vi "Pre Launch Init.vi"(11 "Nested in":refnum<class "Paquetes.lvclass">) -> (0 "error out":errorcluster, 3 "Nested out":refnum<class "Paquetes.lvclass">)   [LabVIEW 2020, in "Paquetes.lvlib" / "Paquetes.lvclass"]
doc: "(<B>Filename</B>: Actor Framework.lvlib:Actor.lvclass:Pre Launch Init.vi)\n\nDefines behavior that occurs after the Launch Nested Actor method is invoked but before the actor's Actor Core method begins running.\n\nBy default, this method does nothing. A descendant class may override it to define behavior."
uses:
  Paquetes.lvclass
  C:/Program Files (x86)/National Instruments/LabVIEW 2020/vi.lib/ActorFramework/Actor/Actor.lvclass
  Paquetes.lvclass/Paquetes.ctl
  <vilib>/ActorFramework/Actor/Actor.lvclass/Actor.ctl
  <vilib>/ActorFramework/Message Enqueuer/Message Enqueuer.lvclass/Message Enqueuer.ctl
  <vilib>/ActorFramework/Message Enqueuer/Enqueue.vi
  <vilib>/ActorFramework/Message Enqueuer/Init from Existing Queue.vi
  Paquetes Messages/DRAW FP PAQUETES IN UI Msg/DRAW FP PAQUETES IN UI Msg.lvclass
  C:/Program Files (x86)/National Instruments/LabVIEW 2020/vi.lib/ActorFramework/Message/Message.lvclass
  <vilib>/ActorFramework/Message Priority Queue/Priority Enqueue.vi
  <vilib>/ActorFramework/Message Enqueuer/Message Enqueuer.lvclass
  <vilib>/ActorFramework/Actor/Actor.lvclass
  C:/Users/HP/Desktop/Salma_Aguayo/Paquetes/Paquetes.lvclass
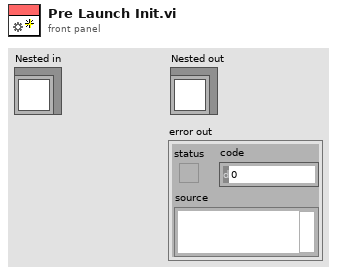
[diagram p1: front panel]
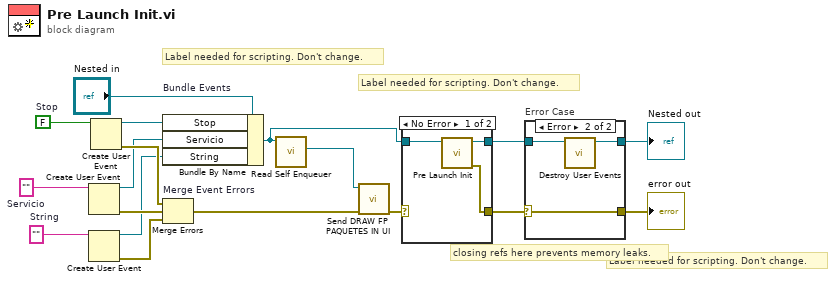
[diagram p0: block diagram]
diagram:
  w3 = ""  # String
  w6 = ""  # Servicio
  w17 = FALSE  # Stop
  # "Label needed for scripting. Don't change."
  # "Label needed for scripting. Don't change."
  # "Label needed for scripting. Don't change."
  # "closing refs here prevents memory leaks."
  n1 = Create User Event(user event datatype=w6) -> (user event=w5:refnum<user-event>, error out=w4:errorcluster)  [unwired: 1 in]
  n2 = Create User Event(user event datatype=w3) -> (user event=w2:refnum<user-event>, error out=w1:errorcluster)  [unwired: 1 in]
  n3 = Create User Event(user event datatype=w17) -> (user event=w14:refnum<user-event>, error out=w16:errorcluster)  [unwired: 1 in]
  n4 = Bundle By Name "Bundle Events"(cluster="Nested in", "Stop"=w14, "Servicio"=w5, "String"=w2) -> (w8:refnum<class "Paquetes.lvclass">)
  n5 = Merge Errors "Merge Event Errors"(w16, w4, w1) -> (w7:errorcluster)
  n6 = call <vilib>:"Read Self Enqueuer.vi"("Actor"=w8) -> ("Self Enqueuer"=w9:refnum<class "Message Enqueuer.lvclass">)  [unwired: 10 in]
  n7 = call "Send DRAW FP PAQUETES IN UI.vi"("error in (no error)"=w7, "Message Enqueuer"=w9) -> ("error out"=w10:errorcluster)  [unwired: 8 in, 1 out]
  n8 = case shown="No Error" w10 {
    selector: w10 -> [_ w23]
    tunnel: [w21 w22] -> w12
    tunnel: w8 -> [w20 w22]
    tunnel: [w19 w23] -> w11
    frame No Error {
      n9 = call-parent "Pre Launch Init.vi"("Actor in"=w20) -> ("error out"=w19:errorcluster, "Actor out"=w21:refnum<class "Paquetes.lvclass">)  [unwired: 9 in]
    }
    frame Error {
    }
  }
  n10 = case "Error Case" shown="Error" w11 {
    selector: w11 -> [w24 w28]
    tunnel: w12 -> [w25 w27]
    tunnel: [w25 w26] -> w15
    tunnel: [w24 w28] -> w13
    frame No Error {
    }
    frame Error {
      n11 = call "Destroy User Events.vi"("UI Template in"=w27) -> ("UI Template out"=w26:refnum<class "Paquetes.lvclass">)  [unwired: 10 in]
    }
  }
  "error out" <- w13
  "Nested out" <- w15
